vi "updateEnumCheckOut.vi"(0 "reference in":refnum<class "Items Controller.lvclass">, 5 "error in (no error)":errorcluster) -> (14 "reference out":refnum<class "Items Controller.lvclass">, 19 "error out":errorcluster)   [LabVIEW 2015, in "Items Controller.lvclass"]
uses:
  Items Controller.lvclass
  APP/excelFile_class/fileType.ctl
  File Controller_llb/File Controller.lvclass
  APP/excelFile_class/excelFile.lvclass
panel:
  in  "target class":refnum<vi>
  in  "target class":refnum<vi>
  in  "target class":refnum<vi>
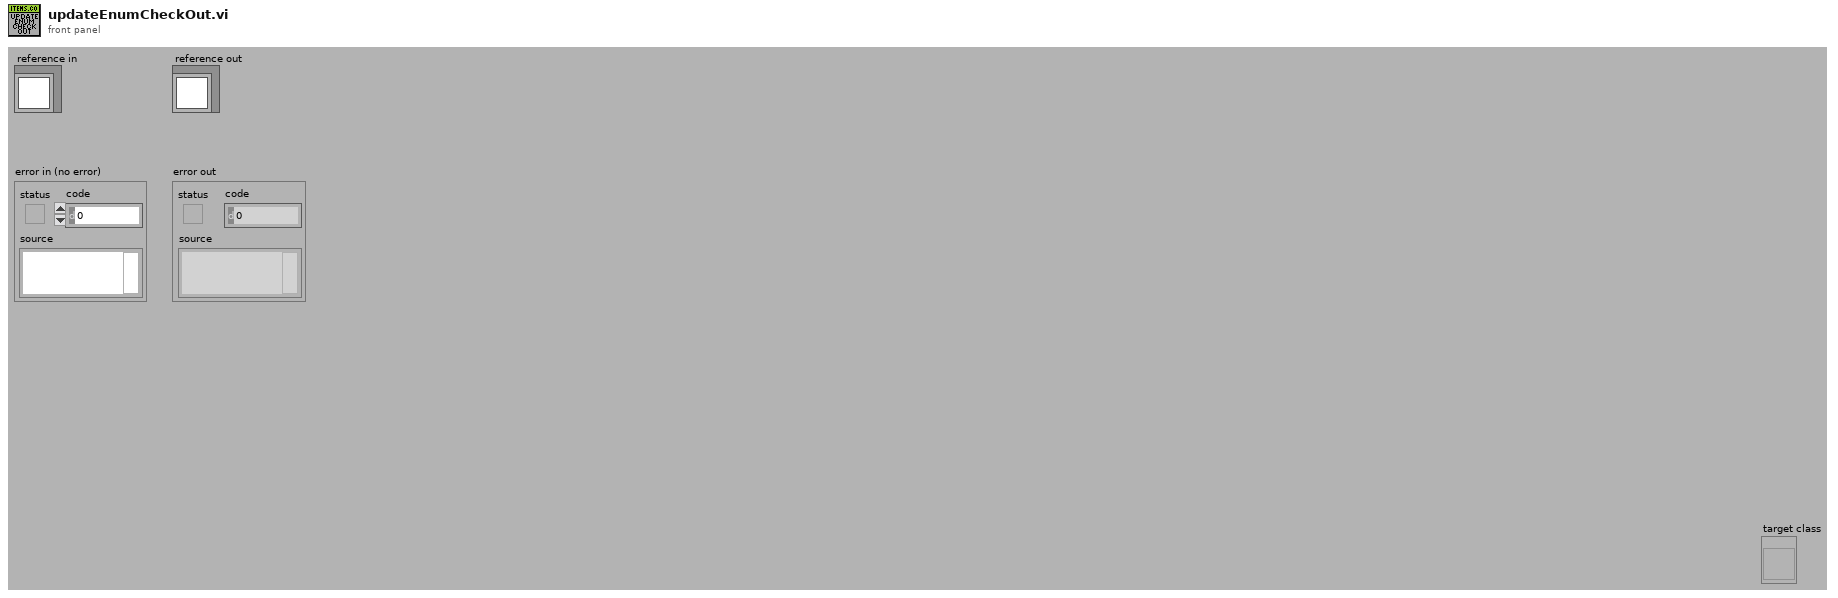
[diagram p1: front panel]
types:
  T1 = typedef "excelFile.lvclass/fileType.ctl" = enum16{"devices", "items", "partsTracking", "TSR"}
  T2 = typedef "Items Controller.lvclass/ObjectAttributesRef.ctl" = refnum<data-value>
  T3 = typedef "Items Controller.lvclass/ObjectAttributes.ctl" = cluster{"MyAttribute":dbl, "data":string[][][], "file_controller_ref":refnum<class "File Controller.lvclass">, "checkIN_ref":refnum<class "checkIN.lvclass">, "checkOUT_ref":refnum<class "checkOUT.lvclass">, "item_ref":refnum<class "item.lvclass">}
  T4 = enum32{"invalid app kind", "Development System", "Run Time System", "Student Edition", "Embedded LabVIEW", "Evaluation", "Custom"}
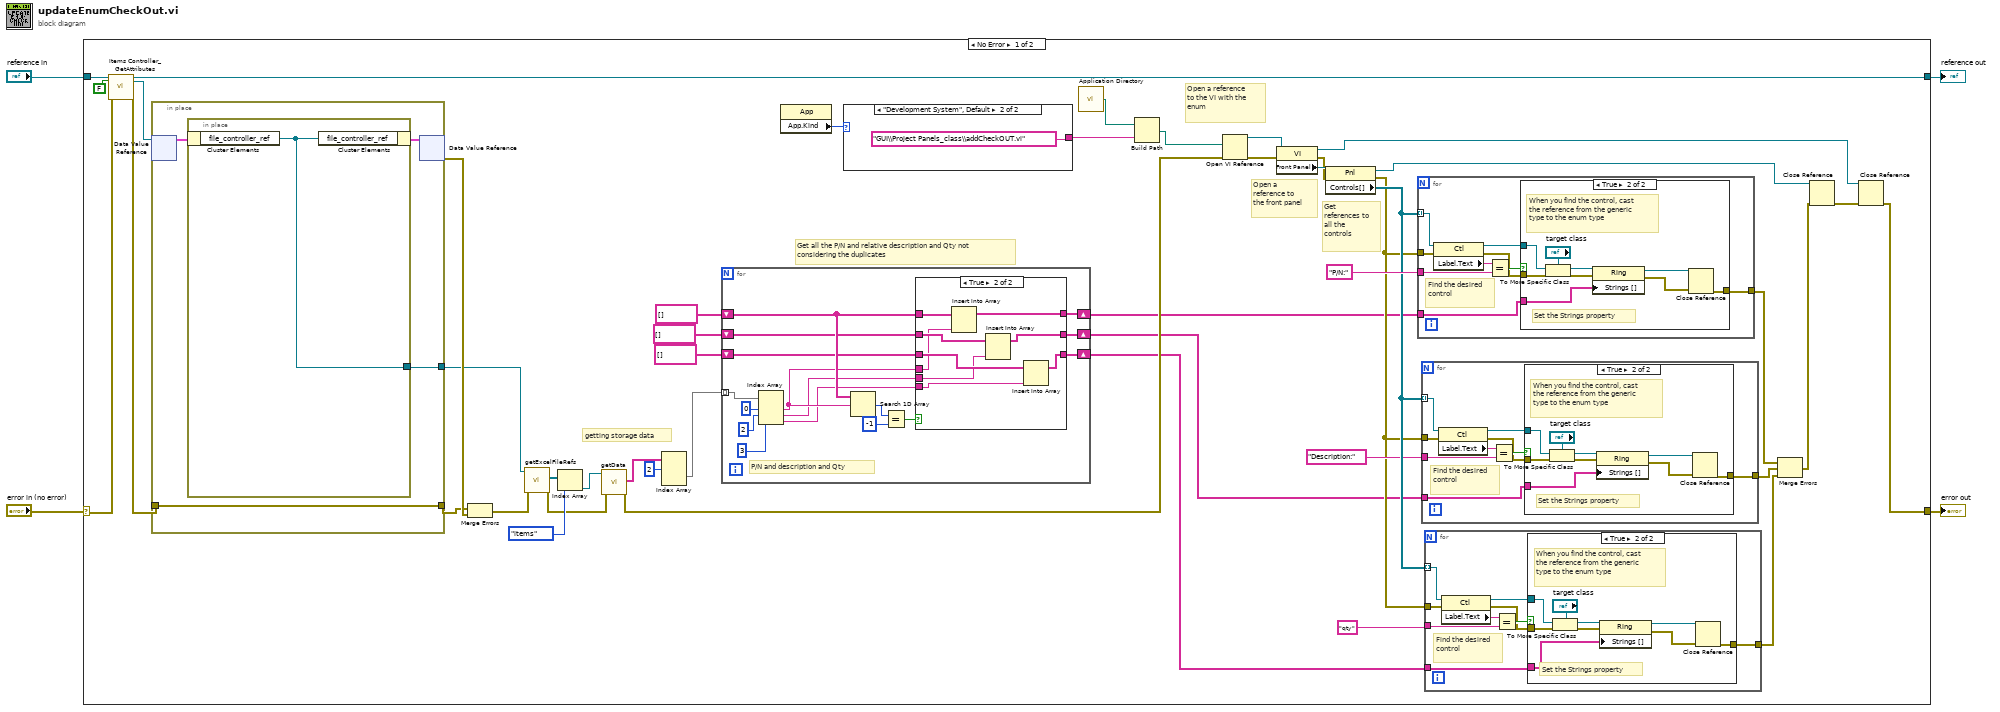
[diagram p0: block diagram]
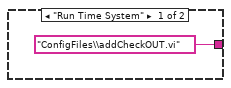
[diagram p2: hidden frame]
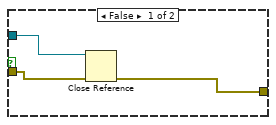
[diagram p3: hidden frame]
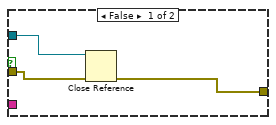
[diagram p4: hidden frame]
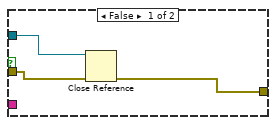
[diagram p5: hidden frame]
diagram:
  n1 = case shown="No Error" "error in (no error)" {
    selector: "error in (no error)" -> [w45 w149]
    tunnel: [w20 w149] -> w3
    tunnel: [w43 w148] -> w1
    tunnel: "reference in" -> [w47 w148]
    frame No Error {
      # "Open a reference to the VI with the enum"
      # "Open a reference to the front panel"
      # "Get references to all the controls"
      # "Get all the P/N and relative description and Qty not\nconsidering the duplicates"
      # "getting storage data"
      n2 = call "Items Controller_GetAttributes.vi"("reference in"=w47, "return data? (T)"=FALSE, "error in (no error)"=w45) -> ("reference out"=w43:refnum<class "Items Controller.lvclass">, "attributes ref"=w42:T2, "error out"=w44:errorcluster)  [unwired: 13 in, 1 out]
      n3 = in-place {
        in-place-border: w44 -> [w144]
        in-place-border: [w144] -> w48
        in-place-border: [w143] -> w40
        n4 = in-place-dvr #1(w42) -> (w145:T3)  [unwired: 1 out]
        n5 = in-place {
          in-place-border: [w147] -> w143
          n6 = in-place-cluster #2(w145) -> ("file_controller_ref"=w147:refnum<class "File Controller.lvclass">)
          n7 = in-place-cluster #2("file_controller_ref"=w147) -> (w146:T3)
        }
        n8 = in-place-dvr #1(w146) -> (w49:errorcluster)  [unwired: 1 out]
      }
      n9 = Merge Errors(w48, w49) -> (w39:errorcluster)
      n10 = call "getExcelFileRefs.vi"("error in (no error)"=w39, "reference in"=w40) -> ("error out"=w36:errorcluster, "excelFile_refs"=w41:refnum<class "excelFile.lvclass">[])  [unwired: 7 in, 1 out]
      n11 = Index Array(array=w41, index=fileType."items" ("fileType")) -> (element=w37:refnum<class "excelFile.lvclass">)
      n12 = call "getData.vi"("error in (no error)"=w36, "reference in"=w37) -> ("error out"=w21:errorcluster, "data"=w35:string[][][])  [unwired: 7 in, 1 out]
      n13 = Index Array(array=w35, index (dim 0)=2 ("index (page)")) -> (element=w33:string[][])  [unwired: 2 in]
      n14 = for {
        tunnel: w33 -> [w130] mode=indexing
        shift-right: [w117] -> w9
        shift-left: string[] [] -> [w123]
        shift-right: [w116] -> w8
        shift-left: string[] [] -> [w122]
        shift-right: [w115] -> w7
        shift-left: string[] [] -> [w121]
        # "P/N and description and Qty"
        n15 = Index Array(array=w130, index #1=0 ("index"), index #2=2 ("index"), index #3=3 ("index")) -> (element #1=w120:string, element #2=w119:string, element #3=w118:string)
        n16 = Search 1D Array(1D array=w123, element=w120) -> (index of element=w125:i32)  [unwired: 1 in]
        n17 = Equal?(x=w125, y=-1) -> (x = y?=w126:bool)
        n18 = case shown="True" w126 {
          tunnel: w123 -> [w133 w142]
          tunnel: w122 -> [w132 w140]
          tunnel: w121 -> [w131 w138]
          tunnel: w120 -> [_ w136]
          tunnel: w119 -> [_ w135]
          tunnel: w118 -> [_ w134]
          tunnel: [w133 w141] -> w117
          tunnel: [w132 w139] -> w116
          tunnel: [w131 w137] -> w115
          frame False {
          }
          frame True {
            n19 = Insert Into Array(array=w142, new element=w136) -> (w141:string[])  [unwired: 1 in]
            n20 = Insert Into Array(array=w140, new element=w135) -> (w139:string[])  [unwired: 1 in]
            n21 = Insert Into Array(array=w138, new element=w134) -> (w137:string[])  [unwired: 1 in]
          }
        }
      }
      n22 = property class="App"() -> ("App.Kind"=w6:T4)  [unwired: 2 in, 2 out]
      n23 = case shown="\"Development System\", Default" w6 {
        tunnel: ["ConfigFiles\\addCheckOUT.vi" ("name or relative path") "GUI\\Project Panels_class\\addCheckOUT.vi" ("name or relative path")] -> w5
        frame "Run Time System" {
        }
        frame "Development System", Default {
        }
      }
      n24 = call <vilib>:"Application Directory.vi"() -> ("Application Directory"=w11:path)
      n25 = Build Path(base path=w11, name or relative path=w5) -> (appended path=w10:path)
      n26 = Open VI Reference(vi path=w10, error in (no error)=w21) -> (vi reference=w29:refnum<vi>, error out=w24:errorcluster)  [unwired: 4 in]
      n27 = property class="VI"(reference=w29, error in=w24) -> (reference out=w27:refnum<vi>, error out=w23:errorcluster, "Front Panel"=w28:refnum<vi>)
      n28 = property class="Pnl"(reference=w28, error in=w23) -> (reference out=w26:refnum<vi>, error out=w17:errorcluster, "Controls[]"=w19:refnum<vi>[])
      n29 = for {
        tunnel: w19 -> [w102] mode=indexing
        tunnel: "P/N:" -> [w100]
        tunnel: w17 -> [w97]
        tunnel: [w95] -> w15
        tunnel: w9 -> [w94]
        # "Find the desired control"
        n30 = property class="Ctl"(reference=w102, error in=w97) -> (reference out=w98:refnum<vi>, error out=w96:errorcluster, "Label.Text"=w101:string)
        n31 = Equal?(x=w101, y=w100) -> (x = y?=w99:bool)
        n32 = case shown="True" w99 {
          tunnel: w98 -> [w105 w114]
          tunnel: w96 -> [w104 w110]
          tunnel: [w103 w107] -> w95
          tunnel: w94 -> [_ w106]
          frame False {
            n33 = Close Reference(reference=w105, error in (no error)=w104) -> (error out=w103:errorcluster)
          }
          frame True {
            # "Set the Strings property"
            # "When you find the control, cast the reference from the generic type to the enum type"
            n34 = To More Specific Class(target class="target class", reference=w114, error in=w110) -> (specific class reference=w112:refnum<vi>, error out=w109:errorcluster)
            n35 = property class="Ring"(reference=w112, error in=w109, "Strings []"=w106) -> (reference out=w111:refnum<vi>, error out=w108:errorcluster)
            n36 = Close Reference(reference=w111, error in (no error)=w108) -> (error out=w107:errorcluster)
          }
        }
      }
      n37 = for {
        tunnel: w19 -> [w81] mode=indexing
        tunnel: "Description:" -> [w79]
        tunnel: w17 -> [w76]
        tunnel: [w74] -> w14
        tunnel: w8 -> [w73]
        # "Find the desired control"
        n38 = property class="Ctl"(reference=w81, error in=w76) -> (reference out=w77:refnum<vi>, error out=w75:errorcluster, "Label.Text"=w80:string)
        n39 = Equal?(x=w80, y=w79) -> (x = y?=w78:bool)
        n40 = case shown="True" w78 {
          tunnel: w77 -> [w84 w93]
          tunnel: w75 -> [w83 w89]
          tunnel: [w82 w86] -> w74
          tunnel: w73 -> [_ w85]
          frame False {
            n41 = Close Reference(reference=w84, error in (no error)=w83) -> (error out=w82:errorcluster)
          }
          frame True {
            # "Set the Strings property"
            # "When you find the control, cast the reference from the generic type to the enum type"
            n42 = To More Specific Class(target class="target class", reference=w93, error in=w89) -> (specific class reference=w91:refnum<vi>, error out=w88:errorcluster)
            n43 = property class="Ring"(reference=w91, error in=w88, "Strings []"=w85) -> (reference out=w90:refnum<vi>, error out=w87:errorcluster)
            n44 = Close Reference(reference=w90, error in (no error)=w87) -> (error out=w86:errorcluster)
          }
        }
      }
      n45 = for {
        tunnel: w19 -> [w60] mode=indexing
        tunnel: "qty" -> [w58]
        tunnel: w17 -> [w55]
        tunnel: [w53] -> w13
        tunnel: w7 -> [w52]
        # "Find the desired control"
        n46 = property class="Ctl"(reference=w60, error in=w55) -> (reference out=w56:refnum<vi>, error out=w54:errorcluster, "Label.Text"=w59:string)
        n47 = Equal?(x=w59, y=w58) -> (x = y?=w57:bool)
        n48 = case shown="True" w57 {
          tunnel: w56 -> [w63 w72]
          tunnel: w54 -> [w62 w68]
          tunnel: [w61 w65] -> w53
          tunnel: w52 -> [_ w64]
          frame False {
            n49 = Close Reference(reference=w63, error in (no error)=w62) -> (error out=w61:errorcluster)
          }
          frame True {
            # "Set the Strings property"
            # "When you find the control, cast the reference from the generic type to the enum type"
            n50 = To More Specific Class(target class="target class", reference=w72, error in=w68) -> (specific class reference=w70:refnum<vi>, error out=w67:errorcluster)
            n51 = property class="Ring"(reference=w70, error in=w67, "Strings []"=w64) -> (reference out=w69:refnum<vi>, error out=w66:errorcluster)
            n52 = Close Reference(reference=w69, error in (no error)=w66) -> (error out=w65:errorcluster)
          }
        }
      }
      n53 = Merge Errors(w15, w14, w13) -> (w12:errorcluster)
      n54 = Close Reference(reference=w26, error in (no error)=w12) -> (error out=w22:errorcluster)
      n55 = Close Reference(reference=w27, error in (no error)=w22) -> (error out=w20:errorcluster)
    }
    frame Error {
    }
  }
  "error out" <- w3
  "reference out" <- w1
